vi "sinefreq.vi"() -> ()   [LabVIEW 2018]
uses:
  <vilib>/DAQmx/write.llb/DAQmx Write (Digital Wfm 1Chan NSamp).vi
  <vilib>/DAQmx/create/channels.llb/DAQmx Create Channel (DO-Digital Output).vi
  <vilib>/Waveform/DWDTOps.llb/DWDT Analog to Digital.vi
  <vilib>/DAQmx/configure/timing.llb/DAQmx Timing (Sample Clock).vi
  <vilib>/Waveform/DWDTOps.llb/DWDT Digital Signal Subset.vi
  <vilib>/Waveform/DWDTOps.llb/DWDT Append Digital Signals.vi
  <vilib>/Waveform/DWDTOps.llb/DWDT Uncompress Digital.vi
  <vilib>/DAQmx/miscellaneous.llb/DAQmx Fill In Error Info.vi
panel:
  out "Shape of pulse 2":digitalwaveform(graph)
  out "time of 1 bit (ms)":dbl
  in  "frequency":dbl=1000.0 format="%0.2f"
  out "Array":u32[](array[numeric])
  out "Digitsl Pulse input":waveform(dbl)(graph)
  in  "Maximum bits":dbl
  in  "Digital pulse shape":dbl[](array[numeric])
  in  "amplitude":dbl
  in  "Steps set in driver":dbl
  in  "stop":bool
  out "number of samples written per channel":u32
  in  "samples per channel":i32=1000
  out "Shape of pulse":digitalwaveform(graph)
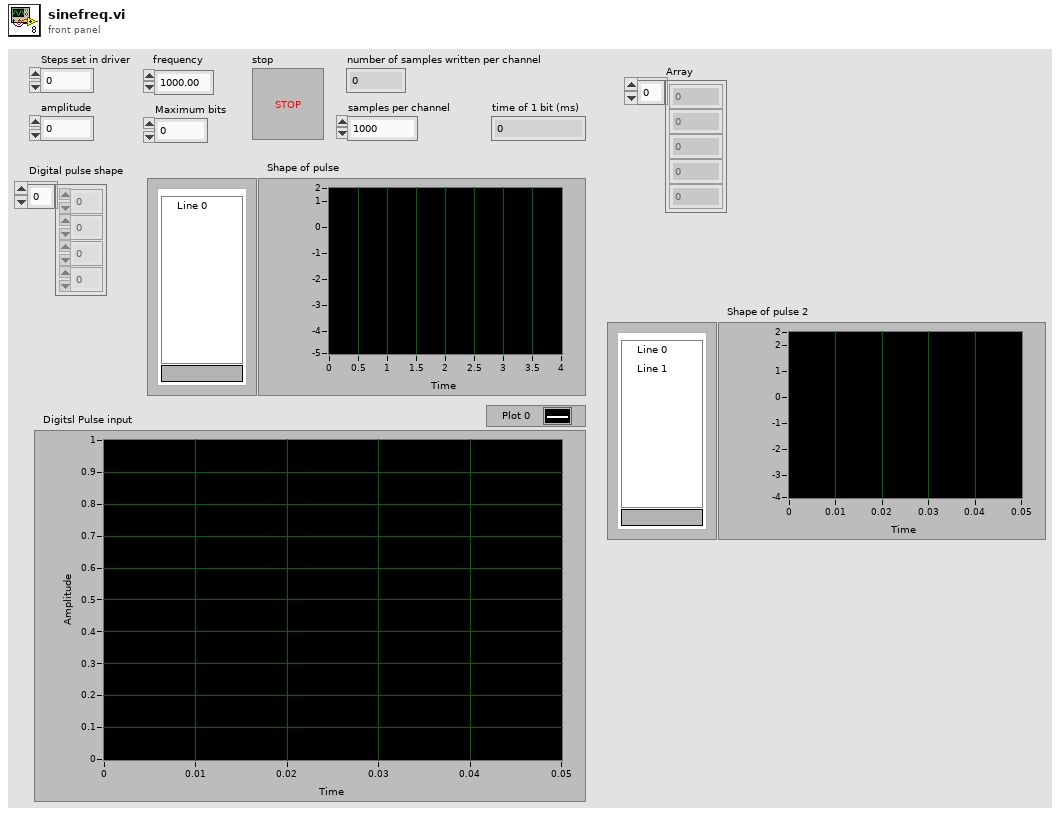
[diagram p1: front panel]
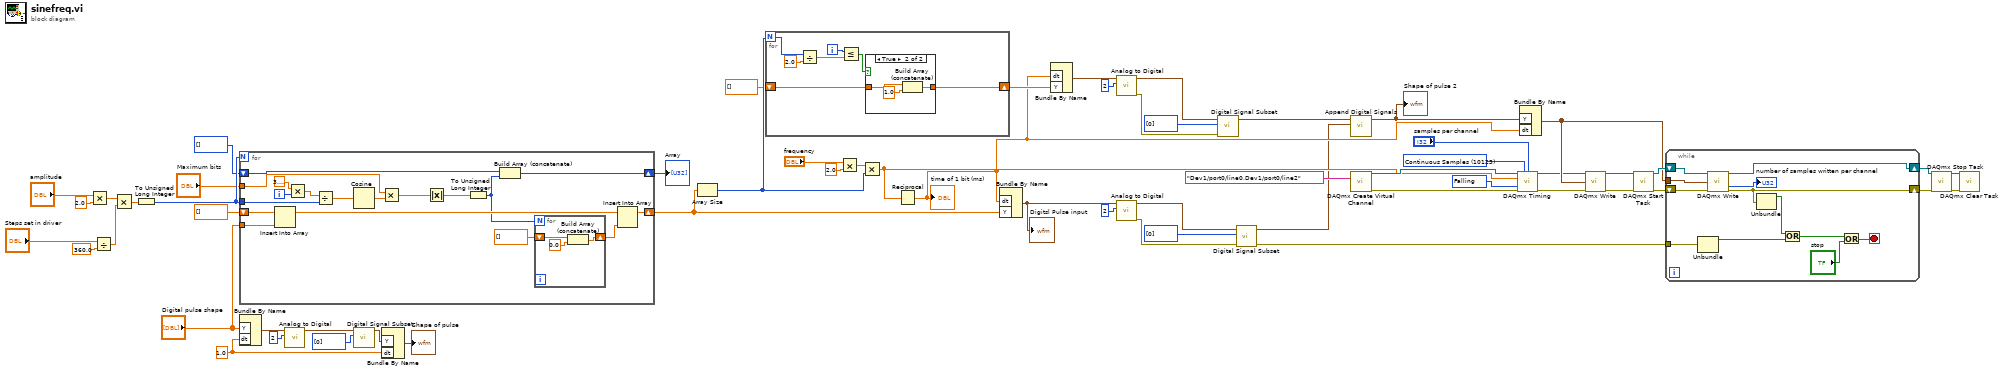
[diagram p0: block diagram]
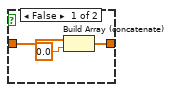
[diagram p2: hidden frame]
diagram:
  w23 = 1.0 ("dt")
  w56 = 10171 items=["Rising"=10280, "Falling"=10171] ("active edge")
  w58 = 10123 items=["Finite Samples"=10178, "Continuous Samples"=10123, "Hardware Timed Single Point"=12522] ("sample mode")
  n1 = Multiply(x="amplitude", y=2.0) -> (x*y=w39:dbl)
  n2 = Divide(x="Steps set in driver", y=360.0) -> (x/y=w46:dbl)
  n3 = Multiply(x=w39, y=w46) -> (x*y=w43:dbl)
  n4 = To Unsigned Long Integer(number=w43) -> (unsigned 32bit integer=w45:u32)
  n5 = for {
    N: w45 -> [_]
    shift-right: [w73] -> w13
    shift-left: dbl[] [] -> [w62]
    tunnel: "Maximum bits" -> [w76]
    tunnel: w45 -> [w66]
    shift-right: [w64] -> w35
    shift-left: u32[] [] -> [w63]
    tunnel: "Digital pulse shape" -> [w61]
    i -> [w69]
    n6 = Insert Into Array(array=w62, new element=w61) -> (w74:dbl[])  [unwired: 1 in]
    n7 = Multiply(x=3.141592653589793, y=w69) -> (x*y=w78:dbl)
    n8 = Divide(x=w78, y=w66) -> (x/y=w77:dbl)
    n9 = Cosine(x=w77) -> (cos(x)=w75:dbl)
    n10 = Multiply(x=w76, y=w75) -> (x*y=w67:dbl)
    n11 = Absolute Value(x=w67) -> (abs(x)=w68:dbl)
    n12 = To Unsigned Long Integer(number=w68) -> (unsigned 32bit integer=w65:u32)
    n13 = Build Array (concatenate)(w63, w65) -> (w64:u32[])
    n14 = for {
      N: w65 -> [_]
      shift-right: [w79] -> w71
      shift-left: dbl[] [] -> [w80]
      n15 = Build Array (concatenate)(w80, 0.0 ("element")) -> (w79:dbl[])
    }
    n16 = Insert Into Array(array=w74, new element=w71) -> (w73:dbl[])  [unwired: 1 in]
  }
  "Array" <- w35
  n17 = Bundle By Name("Y"="Digital pulse shape", "dt"=w23) -> (w26:waveform(dbl))  [unwired: 1 in]
  n18 = call-poly <vilib>:"Analog to Digital.vi"("resolution (16 bit)"=2, "analog waveform"=w26) -> ("digital waveform"=w25:digitalwaveform)  [unwired: 6 in, 3 out]
  n19 = call-poly <vilib>:"Digital Signal Subset.vi"("signals"=i32[] [0], "digital waveform"=w25) -> ("digital subset"=w24:digitalwaveform)  [unwired: 8 in, 1 out]
  n20 = Bundle By Name("Y"=w24, "dt"=w23) -> (→"Shape of pulse":digitalwaveform)  [unwired: 1 in]
  n21 = Array Size(array=w13) -> (size(s)=w15:i32)
  n22 = for {
    N: w15 -> [w85]
    shift-right: [w83] -> w12
    shift-left: dbl[] [] -> [w82]
    i -> [w87]
    n23 = Divide(x=w85, y=2.0) -> (x/y=w84:dbl)
    n24 = Less Or Equal?(x=w87, y=w84) -> (x <= y?=w88:bool)
    n25 = case shown="True" w88 {
      tunnel: [w89 w94] -> w83
      tunnel: w82 -> [w90 w93]
      frame False {
        n26 = Build Array (concatenate)(w90, 0.0 ("element")) -> (w89:dbl[])
      }
      frame True {
        n27 = Build Array (concatenate)(w93, 1.0 ("element")) -> (w94:dbl[])
      }
    }
  }
  n28 = Multiply(x="frequency", y=2.0) -> (x*y=w30:dbl)
  n29 = Multiply(x=w30, y=w15) -> (x*y=w17:dbl)
  n30 = Reciprocal(x=w17) -> (1/x=w11:dbl)
  "time of 1 bit (ms)" <- w11
  n31 = Bundle By Name("dt"=w11, "Y"=w13) -> (w32:waveform(dbl))  [unwired: 1 in]
  "Digitsl Pulse input" <- w32
  n32 = Bundle By Name("dt"=w11, "Y"=w12) -> (w10:waveform(dbl))  [unwired: 1 in]
  n33 = call-poly <vilib>:"Analog to Digital.vi"("resolution (16 bit)"=2, "analog waveform"=w10) -> ("error out"=w7:errorcluster, "digital waveform"=w5:digitalwaveform)  [unwired: 6 in, 2 out]
  n34 = call-poly <vilib>:"Analog to Digital.vi"("resolution (16 bit)"=2, "analog waveform"=w32) -> ("error out"=w34:errorcluster, "digital waveform"=w4:digitalwaveform)  [unwired: 6 in, 2 out]
  n35 = call-poly <vilib>:"Digital Signal Subset.vi"("error in (no error)"=w7, "signals"=i32[] [0], "digital waveform"=w5) -> ("digital subset"=w2:digitalwaveform)  [unwired: 7 in, 1 out]
  n36 = call-poly <vilib>:"Digital Signal Subset.vi"("error in (no error)"=w34, "signals"=i32[] [0], "digital waveform"=w4) -> ("error out"=w33:errorcluster, "digital subset"=w1:digitalwaveform)  [unwired: 7 in]
  n37 = call-poly <vilib>:"Append Digital Signals.vi"("digital waveform (low bits)"=w1, "digital waveform (high bits)"=w2) -> ("digital waveform out"=w3:digitalwaveform)  [unwired: 8 in, 1 out]
  "Shape of pulse 2" <- w3
  n38 = call-poly <vilib>:"DAQmx Create Virtual Channel.vi"("lines"=tag "Dev1/port0/line0,Dev1/port0/line2") -> ("task out"=w59:refnum<k21>, "error out"=w55:errorcluster)  [unwired: 13 in]
  n39 = call-poly <vilib>:"DAQmx Timing.vi"("task/channels in"=w59, "sample mode"=w58, "samples per channel"="samples per channel", "rate"=w17, "active edge"=w56, "error in"=w55) -> ("task out"=w19:refnum<k21>, "error out"=w18:errorcluster)  [unwired: 8 in]
  n40 = Bundle By Name("Y"=w3, "dt"=w11) -> (w28:digitalwaveform)  [unwired: 1 in]
  n41 = call-poly <vilib>:"DAQmx Write.vi"("task/channels in"=w19, "data"=w28, "error in"=w18) -> ("task out"=w47:refnum<k21>, "error out"=w48:errorcluster)  [unwired: 10 in, 1 out]
  n42 = call <vilib>:"DAQmx Start Task.vi"("task/channels in"=w47, "error in"=w48) -> ("task out"=w52:refnum<k21>, "error out"=w49:errorcluster)  [unwired: 12 in]
  n43 = while {
    tunnel: w28 -> [w105]
    shift-right: [w103] -> w51
    shift-left: w52 -> [w104]
    shift-right: [w101] -> w50
    shift-left: w49 -> [w102]
    tunnel: w33 -> [w97]
    stop <- w99 stop-if-true
    n44 = Unbundle(w97) -> ("status"=w96:bool)  [unwired: 2 out]
    n45 = call-poly <vilib>:"DAQmx Write.vi"("task/channels in"=w104, "data"=w105, "error in"=w102) -> ("task out"=w103:refnum<k21>, "number of samples written per channel"=→"number of samples written per channel":u32, "error out"=w101:errorcluster)  [unwired: 10 in]
    n46 = Unbundle(w101) -> ("status"=w98:bool)  [unwired: 2 out]
    n47 = Or(x=w98, y=w96) -> (x .or. y?=w95:bool)
    n48 = Or(x=w95, y="stop") -> (x .or. y?=w99:bool)
  }
  n49 = call <vilib>:"DAQmx Stop Task.vi"("task/channels in"=w51, "error in"=w50) -> ("task out"=w54:refnum<k21>, "error out"=w53:errorcluster)  [unwired: 12 in]
  n50 = call <vilib>:"DAQmx Clear Task.vi"("task in"=w54, "error in"=w53) -> ()  [unwired: 13 in, 1 out]
